vi "main_flow.vi"() -> ()   [LabVIEW 2022 SP3]
uses:
  D:/UOM/EE2044 - Electrical Measurements and Instrumentation/Project/Measurment Project/Quaxo_MQTT_LabVIEW-master/Controls/Connection_Return_Codes.ctl
  D:/UOM/EE2044 - Electrical Measurements and Instrumentation/Project/Measurment Project/Quaxo_MQTT_LabVIEW-master/Controls/QoS.ctl
  D:/UOM/EE2044 - Electrical Measurements and Instrumentation/Project/Measurment Project/Quaxo_MQTT_LabVIEW-master/Controls/Retain_Flag.ctl
  D:/UOM/EE2044 - Electrical Measurements and Instrumentation/Project/Measurment Project/Quaxo_MQTT_LabVIEW-master/Controls/DUP_Flag.ctl
  D:/UOM/EE2044 - Electrical Measurements and Instrumentation/Project/Measurment Project/Quaxo_MQTT_LabVIEW-master/Controls/Connect_Flags.ctl
  D:/UOM/EE2044 - Electrical Measurements and Instrumentation/Project/Measurment Project/Quaxo_MQTT_LabVIEW-master/Controls/User_Info.ctl
  <vilib>/DAQmx/write.llb/DAQmx Write (Digital Bool 1Line 1Point).vi
  <vilib>/DAQmx/read.llb/DAQmx Read (Digital Bool 1Line 1Point).vi
  <vilib>/DAQmx/read.llb/DAQmx Read (Analog 1D DBL NChan 1Samp).vi
  <vilib>/DAQmx/create/channels.llb/DAQmx Create Channel (AI-Voltage-Basic).vi
  <vilib>/DAQmx/create/channels.llb/DAQmx Create Channel (DO-Digital Output).vi
  <vilib>/DAQmx/create/channels.llb/DAQmx Create Channel (DI-Digital Input).vi
  <vilib>/DAQmx/miscellaneous.llb/DAQmx Fill In Error Info.vi
  D:/UOM/EE2044 - Electrical Measurements and Instrumentation/Project/Measurment Project/Quaxo_MQTT_LabVIEW-master/MQTT_Functions.lvlib
panel:
  out "Current":dbl(knob) caption="Current (A)" scale=0.0..5.0
  out "Energy":dbl caption="Energy( VA )"
  in  "clock stop":bool
  out "Time":string
  out "Servo Angle":dbl(knob) scale=0.0..150.0
  in  "stop (F)":bool
  out "PWM Wave":dynamicdata(graph) caption="Square"
  in  "Frequency":dbl=50.0
  in  "Offset":dbl=2.5
  in  "Amplitude":dbl=2.5
  in  "MQTT Broker":cluster{"address (IP)":string, "port":u16}={"address (IP)"="broker.mqttdashboard.com", "port"=1883}
  out "Counter":dbl
  out "OUT COUNT":dbl
  out "IN COUNT":dbl
  in  "Mode":dbl
  in  "Relay 2":tag
  in  "Relay 1":tag
  in  "UP DOWN 2":tag
  in  "UP DOWN 1":tag
  in  "Buzzer":tag
  in  "Door IR 1 & 2 & LDR & Current":tag
  out "LDR Value":dbl(knob) scale=0.0..5.0
  in  "Trigger Period(sec)":dbl
  out "?":bool
  out "?":bool
  out "?":bool
  in  "mqtt stop":bool
  in  "Publish Meta":cluster{"QoS":T1, "Retain":T2, "DUP":T3}
  out "Connection Status":T4=enum."Connection refused: not authorized"
  in  "Client ID":string="NodeE-12345"
  out "Current Time":dbl
  in  "stop":bool
  # "Channel Configure"
  # "MQTT Configure"
  # "MQTT publish interval\nset MQTT Server \nset channels\nset check mode trigger period"
  # "Dev1/ai4:7"
  # "Dev1/port0/line2"
  # "Dev1/port0/line1"
  # "broker.mqtt.cool"
  # "Dev1/port0/line0"
  # "Dev1/port0/line3"
  # "Servo Motor Controller"
  # "Energy Calculation"
  # "Dev1/port0/line4"
  # "Counter Status"
  # "Light Mode"
  # "Low"
  # "Medium"
  # "High"
  # "This Indicate the status of light mode in the room"
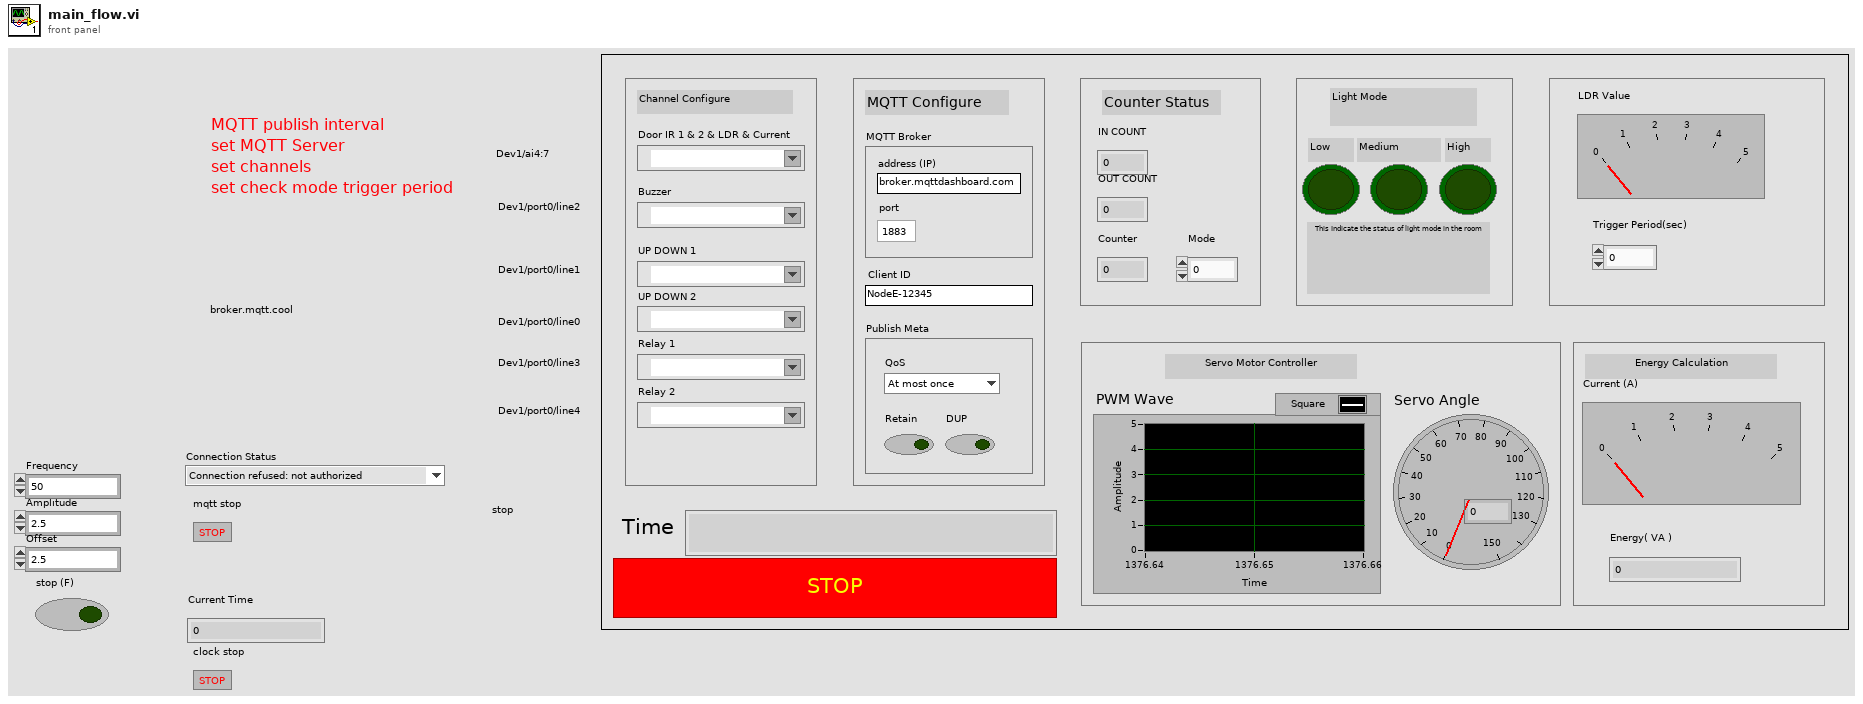
[diagram p1: front panel]
types:
  T1 = typedef "MQTT_Functions.lvlib/QoS.ctl" = enum8{"At most once", "At least once", "Exactly once", "Reserved"}
  T2 = typedef "MQTT_Functions.lvlib/Retain_Flag.ctl" = bool
  T3 = typedef "MQTT_Functions.lvlib/DUP_Flag.ctl" = bool
  T4 = typedef "MQTT_Functions.lvlib/Connection_Return_Codes.ctl" = enum16{"Connection accepted", "Connection refused: unacceptable protocol version", "Connection refused: identifier rejected", "Connection refused: Server unavailable", "Connection refused: bad user name or password", "Connection refused: not authorized"}
  T5 = typedef "MQTT_Functions.lvlib/User_Info.ctl" = cluster{"User Name":string, "Password":string}
  T6 = typedef "MQTT_Functions.lvlib/Connect_Flags.ctl" = cluster{"user name":bool, "password":bool, "will retain":bool, "will flag":bool, "clean session":bool, "reserved":bool, "will QoS":T1}
  T7 = cluster{"QoS":T1, "DUP":T3, "Retain":T2, "Keep Alive (sec)":u16}
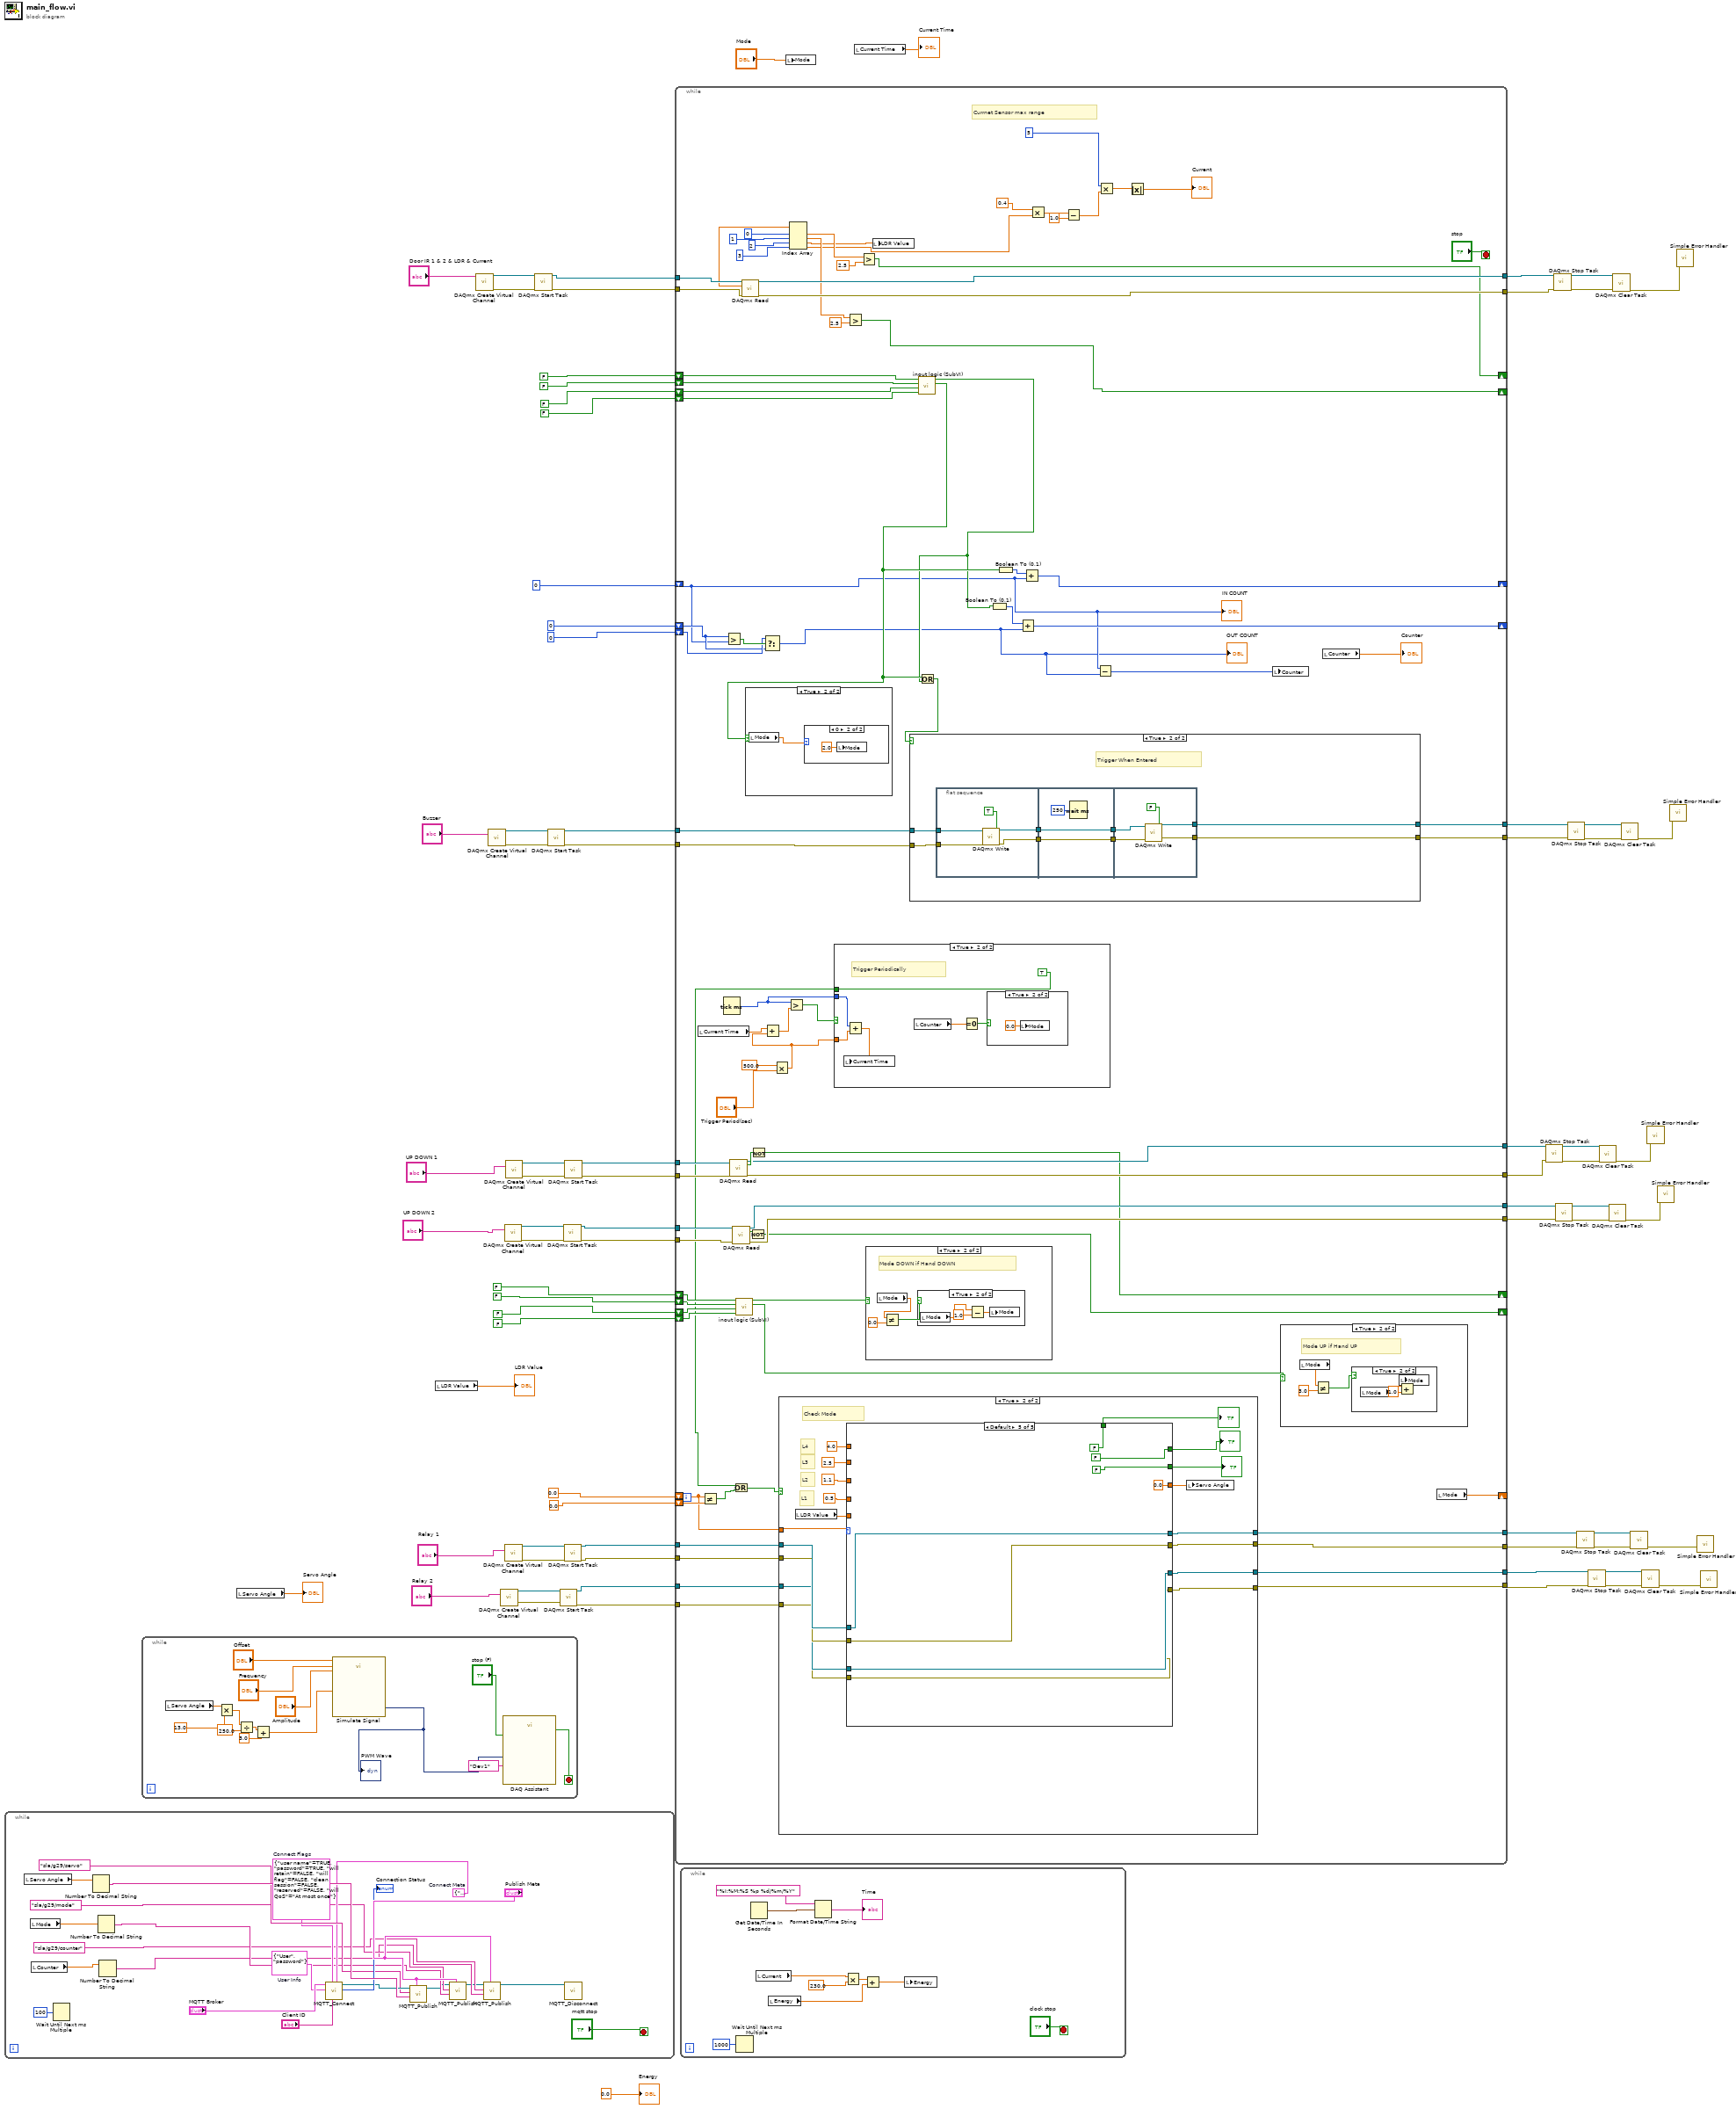
[diagram p0: block diagram]
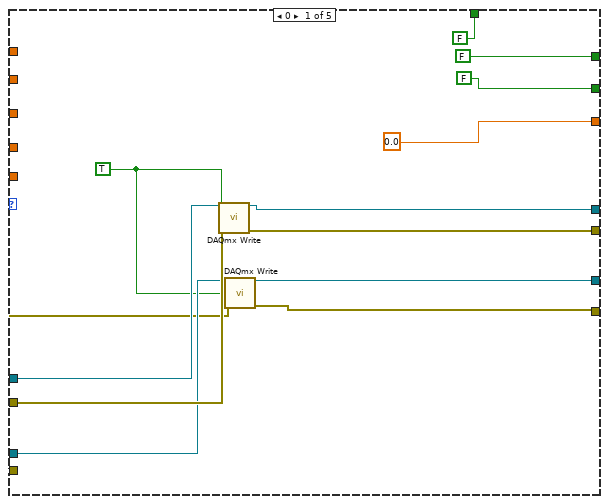
[diagram p5: hidden frame]
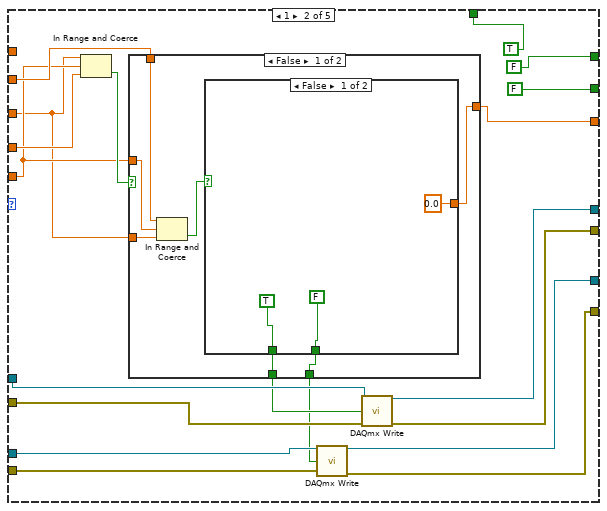
[diagram p6: hidden frame]
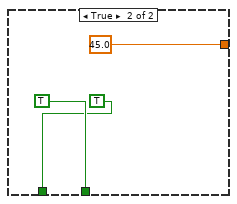
[diagram p7: hidden frame]
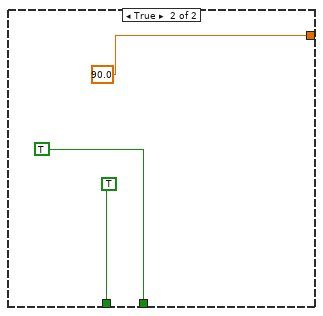
[diagram p8: hidden frame]
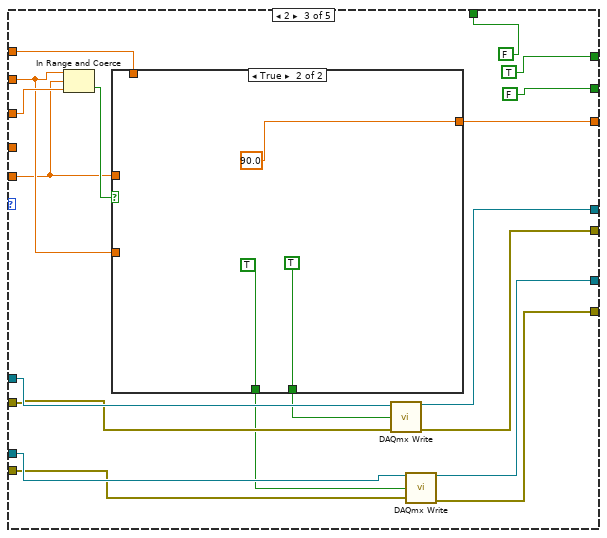
[diagram p9: hidden frame]
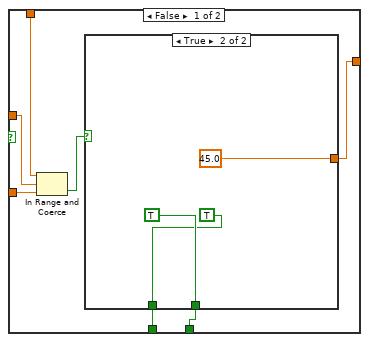
[diagram p10: hidden frame]
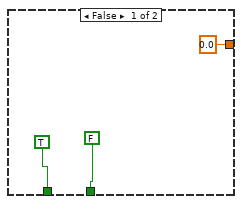
[diagram p11: hidden frame]
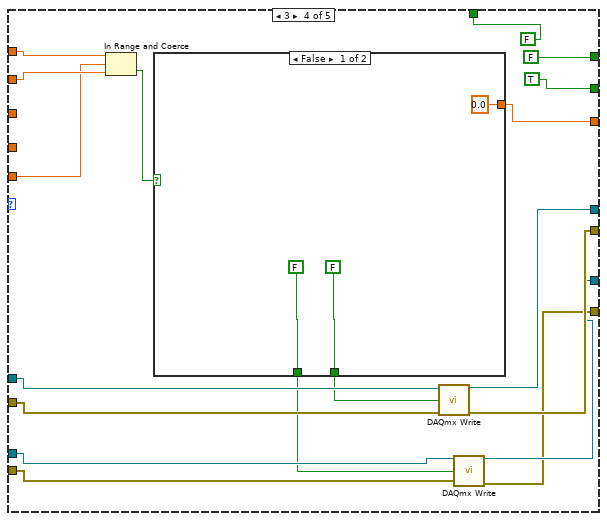
[diagram p12: hidden frame]
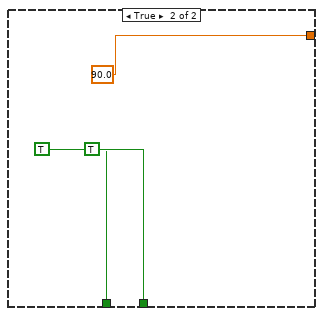
[diagram p13: hidden frame]
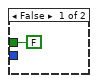
[diagram p18: hidden frame]
diagram:
  n1 = while {
    stop <- "mqtt stop" stop-if-true
    w86 = T5 {"User Name"="User", "Password"="password"}  # User Info
    w87 = T6 {"user name"=TRUE, "password"=TRUE, "will retain"=FALSE, "will flag"=FALSE, "clean session"=FALSE, "reserved"=FALSE, "will QoS"=enum."At most once"}  # Connect Flags
    w88 = T7 {"QoS"=enum."At most once", "DUP"=FALSE, "Retain"=FALSE, "Keep Alive (sec)"=60}  # Connect Meta
    n2 = local read "Servo Angle"() -> (w97:dbl)
    n3 = local read "Mode"() -> (w99:dbl)
    n4 = local read "Counter"() -> (w98:dbl)
    n5 = Wait Until Next ms Multiple(millisecond multiple=u32 100) -> ()  [unwired: 1 out]
    n6 = Number To Decimal String(number=w97) -> (decimal integer string=w96:string)  [unwired: 1 in]
    n7 = Number To Decimal String(number=w99) -> (decimal integer string=w85:string)  [unwired: 1 in]
    n8 = Number To Decimal String(number=w98) -> (decimal integer string=w83:string)  [unwired: 1 in]
    n9 = call "MQTT_Connect.vi"("Connect Meta"=w88, "Client ID"="Client ID", "Connect Flags"=w87, "User Info"=w86, "MQTT Broker"="MQTT Broker") -> ("Connection Status"=→"Connection Status":T4, "connection ID out"=w93:refnum<k5>)  [unwired: 4 in, 1 out]
    n10 = call "MQTT_Publish.vi"("Publish Meta"="Publish Meta", "Message to be published"=w96, "Topic"="sla/g29/servo", "connection ID"=w93) -> ("connection ID out"=w80:refnum<k5>)  [unwired: 6 in, 1 out]
    n11 = call "MQTT_Publish.vi"("Publish Meta"="Publish Meta", "Message to be published"=w85, "Topic"="sla/g29/mode", "connection ID"=w80) -> ("connection ID out"=w79:refnum<k5>)  [unwired: 6 in, 1 out]
    n12 = call "MQTT_Publish.vi"("Publish Meta"="Publish Meta", "Message to be published"=w83, "Topic"="sla/g29/counter", "connection ID"=w79) -> ("connection ID out"=w91:refnum<k5>)  [unwired: 6 in, 1 out]
    n13 = call "MQTT_Disconnect.vi"("connection ID"=w91) -> ()  [unwired: 10 in, 1 out]
  }
  n14 = while {
    stop <- w113 stop-if-true
    n15 = local read "Servo Angle"() -> (w101:dbl)
    n16 = Multiply(x=w101, y=13.0) -> (x*y=w107:dbl)
    n17 = Divide(x=w107, y=250.0) -> (x/y=w106:dbl)
    n18 = Add(x=w106, y=3.0) -> (x+y=w102:dbl)
    n19 = call "Simulate Signal"("Offset"="Offset", "Duty Cycle (%)"=w102, "Frequency"="Frequency", "Amplitude"="Amplitude") -> ("Square"=w109:dynamicdata)  [unwired: 10 in, 1 out]
    "PWM Wave" <- w109
    n20 = call "DAQ Assistant"("data"=w109, "stop (F)"="stop (F)", "device name"=tag "Dev1") -> ("stopped"=w113:bool)  [unwired: 14 in, 2 out]
  }
  n21 = local read "Servo Angle"() -> (→"Servo Angle":dbl)
  n22 = local read "LDR Value"() -> (→"LDR Value":dbl)
  n23 = call-poly <vilib>:"DAQmx Create Virtual Channel.vi"("physical channels"="Door IR 1 & 2 & LDR & Current") -> ("task out"=w74:refnum<k21>, "error out"=w71:errorcluster)  [unwired: 13 in]
  n24 = call-poly <vilib>:"DAQmx Create Virtual Channel.vi"("lines"="Buzzer") -> ("task out"=w59:refnum<k21>, "error out"=w57:errorcluster)  [unwired: 13 in]
  n25 = call-poly <vilib>:"DAQmx Create Virtual Channel.vi"("lines"="Relay 2") -> ("task out"=w20:refnum<k21>, "error out"=w19:errorcluster)  [unwired: 13 in]
  n26 = call-poly <vilib>:"DAQmx Create Virtual Channel.vi"("lines"="UP DOWN 2") -> ("task out"=w48:refnum<k21>, "error out"=w46:errorcluster)  [unwired: 13 in]
  n27 = call-poly <vilib>:"DAQmx Create Virtual Channel.vi"("lines"="Relay 1") -> ("task out"=w23:refnum<k21>, "error out"=w22:errorcluster)  [unwired: 13 in]
  n28 = call-poly <vilib>:"DAQmx Create Virtual Channel.vi"("lines"="UP DOWN 1") -> ("task out"=w49:refnum<k21>, "error out"=w47:errorcluster)  [unwired: 13 in]
  n29 = call <vilib>:"DAQmx Start Task.vi"("task/channels in"=w74, "error in"=w71) -> ("task out"=w72:refnum<k21>, "error out"=w70:errorcluster)  [unwired: 12 in]
  n30 = call <vilib>:"DAQmx Start Task.vi"("task/channels in"=w59, "error in"=w57) -> ("task out"=w56:refnum<k21>, "error out"=w55:errorcluster)  [unwired: 12 in]
  n31 = call <vilib>:"DAQmx Start Task.vi"("task/channels in"=w20, "error in"=w19) -> ("task out"=w15:refnum<k21>, "error out"=w14:errorcluster)  [unwired: 12 in]
  n32 = call <vilib>:"DAQmx Start Task.vi"("task/channels in"=w48, "error in"=w46) -> ("task out"=w41:refnum<k21>, "error out"=w40:errorcluster)  [unwired: 12 in]
  n33 = call <vilib>:"DAQmx Start Task.vi"("task/channels in"=w23, "error in"=w22) -> ("task out"=w17:refnum<k21>, "error out"=w16:errorcluster)  [unwired: 12 in]
  n34 = call <vilib>:"DAQmx Start Task.vi"("task/channels in"=w49, "error in"=w47) -> ("task out"=w43:refnum<k21>, "error out"=w42:errorcluster)  [unwired: 12 in]
  n35 = while {
    shift-right: [w192] -> _
    shift-left: 0.0 ("Mode") -> [w190]
    shift-left: 0.0 ("Mode") -> [w191]
    tunnel: w72 -> [w187]
    tunnel: w70 -> [w186]
    tunnel: [w185] -> w69
    tunnel: [w184] -> w68
    shift-right: [w116] -> _
    shift-left: FALSE -> [w183]
    shift-left: FALSE -> [w182]
    shift-right: [w115] -> _
    shift-left: FALSE -> [w181]
    shift-left: FALSE -> [w156]
    shift-right: [w180] -> _
    shift-left: 0 -> [w118]
    shift-right: [w179] -> _
    shift-left: 0 -> [w119]
    tunnel: w56 -> [w176]
    tunnel: w55 -> [w175]
    tunnel: [w174] -> w51
    tunnel: [w173] -> w50
    shift-right: [w162] -> _
    shift-left: FALSE -> [w160]
    shift-right: [w161] -> _
    shift-left: FALSE -> [w158]
    shift-left: FALSE -> [w159]
    shift-left: FALSE -> [w157]
    tunnel: w43 -> [w170]
    tunnel: w42 -> [w169]
    tunnel: w41 -> [w168]
    tunnel: w40 -> [w167]
    tunnel: [w166] -> w33
    tunnel: [w165] -> w32
    tunnel: [w164] -> w31
    tunnel: [w163] -> w30
    tunnel: w17 -> [w141]
    tunnel: w16 -> [w140]
    tunnel: w15 -> [w139]
    tunnel: w14 -> [w138]
    tunnel: [w137] -> w7
    tunnel: [w136] -> w6
    tunnel: [w135] -> w5
    tunnel: [w134] -> w4
    shift-left: 0 -> [w120]
    stop <- "stop" stop-if-true
    # "Currnet Sensor max range"
    n36 = local read "Current Time"() -> (w199:dbl)
    n37 = Not Equal?(x=w190, y=w191) -> (x != y?=w133:bool)
    n38 = Tick Count (ms)() -> (millisecond timer value=w197:u32)
    n39 = Greater?(x=w119, y=w118) -> (0:w121:bool)
    n40 = call-poly <vilib>:"DAQmx Read.vi"("task/channels in"=w170, "error in"=w169) -> ("task out"=w166:refnum<k21>, "data"=w172:bool, "error out"=w165:errorcluster)  [unwired: 11 in]
    n41 = call-poly <vilib>:"DAQmx Read.vi"("task/channels in"=w168, "error in"=w167) -> ("task out"=w164:refnum<k21>, "data"=w171:bool, "error out"=w163:errorcluster)  [unwired: 11 in]
    n42 = call "inout logic (SubVI).vi"("Sensor 2 (T-2)"=w157, "Sensor 2 (T-1)"=w158, "Sensor 1 (T-2)"=w159, "Sensor 1 (T-1)"=w160) -> ("IN"=w155:bool, "OUT"=w154:bool)  [unwired: 6 in]
    n43 = call-poly <vilib>:"DAQmx Read.vi"("task/channels in"=w187, "error in"=w186) -> ("task out"=w185:refnum<k21>, "data"=w151:dbl[], "error out"=w184:errorcluster)  [unwired: 11 in]
    n44 = Not(x=w171) -> (.not. x?=w161:bool)
    n45 = Not(x=w172) -> (.not. x?=w162:bool)
    n46 = Select(t=w120, s=w121, f=w119) -> (s? t:f=w117:i32)
    "OUT COUNT" <- w117
    n47 = Multiply(x=500.0, y="Trigger Period(sec)") -> (x*y=w193:dbl)
    n48 = Add(x=w199, y=w193) -> (x+y=w196:dbl)
    n49 = Greater?(x=w197, y=w196) -> (0:w198:bool)
    n50 = Index Array(array=w151, index #1=0 ("index"), index #2=1 ("index"), index #3=2 ("index"), index #4=3 ("index")) -> (element #1=w150:dbl, element #2=w147:dbl, element #3=w142:dbl, element #4=w124:dbl)
    n51 = case shown="True" w198 {
      tunnel: w197 -> [_ w357]
      tunnel: w193 -> [_ w356]
      tunnel: [FALSE ("Check") TRUE ("Check")] -> w131
      frame False {
      }
      frame True {
        # "Trigger Periodically"
        n52 = Add(x=w357, y=w356) -> (x+y=w358:dbl)
        n53 = local write "Current Time"(w358) -> ()
        n54 = local read "Counter"() -> (w355:dbl)
        n55 = Equal To 0?(x=w355) -> (x = 0?=w354:bool)
        n56 = case shown="True" w354 {
          frame False {
          }
          frame True {
            n57 = local write "Mode"(0.0 ("Mode")) -> ()
          }
        }
      }
    }
    n58 = Or(x=w131, y=w133) -> (x .or. y?=w132:bool)
    n59 = case shown="True" w132 {
      tunnel: w190 -> [_ w224]
      tunnel: w141 -> [w206 w223]
      tunnel: w140 -> [w205 w222]
      tunnel: w139 -> [w204 w221]
      tunnel: w138 -> [w203 w220]
      tunnel: [w206 w219] -> w137
      tunnel: [w205 w218] -> w136
      tunnel: [w204 w217] -> w135
      tunnel: [w203 w216] -> w134
      frame False {
      }
      frame True {
        # "L4"
        # "L1"
        # "L3"
        # "L2"
        # "Check Mode"
        n60 = local read "LDR Value"() -> (w214:dbl)
        n61 = case shown="Default" w224 {
          tunnel: w223 -> [w237 w256 w291 w325 w339]
          tunnel: w222 -> [w236 w254 w290 w324 w338]
          tunnel: w221 -> [w235 w252 w289 w323 w337]
          tunnel: w220 -> [w234 w250 w288 w322 w336]
          tunnel: [w233 w255 w287 w321 w339] -> w219
          tunnel: [w232 w253 w286 w320 w338] -> w218
          tunnel: [w231 w251 w285 w319 w337] -> w217
          tunnel: [w230 w249 w284 w318 w336] -> w216
          tunnel: 1.1 -> [_ w244 w283 _ _]
          tunnel: 0.5 -> [_ w247 _ _ _]
          tunnel: w214 -> [_ w245 w276 w314 _]
          tunnel: 2.5 -> [_ w246 w277 w315 _]
          tunnel: 4.0 -> [_ _ w278 w316 _]
          tunnel: [0.0 ("Servo Angle") w241 w281 w313 0.0 ("A")] -> w210
          tunnel: [FALSE TRUE FALSE FALSE FALSE] -> w209
          tunnel: [FALSE FALSE TRUE FALSE FALSE] -> w208
          tunnel: [FALSE FALSE FALSE TRUE FALSE] -> w207
          frame 0 {
            w229 = TRUE ("data")
            n62 = call-poly <vilib>:"DAQmx Write.vi"("task/channels in"=w237, "data"=w229, "error in"=w236) -> ("task out"=w233:refnum<k21>, "error out"=w232:errorcluster)  [unwired: 10 in, 1 out]
            n63 = call-poly <vilib>:"DAQmx Write.vi"("task/channels in"=w235, "data"=w229, "error in"=w234) -> ("task out"=w231:refnum<k21>, "error out"=w230:errorcluster)  [unwired: 10 in, 1 out]
          }
          frame 1 {
            n64 = In Range and Coerce(upper limit=w244, x=w245, lower limit=w247) -> (In Range?=w248:bool)  [unwired: 1 out]
            n65 = case shown="False" w248 {
              tunnel: [w259 90.0] -> w241
              tunnel: [w258 TRUE] -> w242
              tunnel: [w257 TRUE] -> w243
              tunnel: w246 -> [w263 _]
              tunnel: w244 -> [w262 _]
              tunnel: w245 -> [w261 _]
              frame False {
                n66 = In Range and Coerce(upper limit=w263, x=w261, lower limit=w262) -> (In Range?=w260:bool)  [unwired: 1 out]
                n67 = case shown="False" w260 {
                  tunnel: [0.0 45.0] -> w259
                  tunnel: [FALSE TRUE] -> w258
                  tunnel: [TRUE TRUE] -> w257
                  frame False {
                  }
                  frame True {
                  }
                }
              }
              frame True {
              }
            }
            n68 = call-poly <vilib>:"DAQmx Write.vi"("task/channels in"=w252, "data"=w242, "error in"=w250) -> ("task out"=w251:refnum<k21>, "error out"=w249:errorcluster)  [unwired: 10 in, 1 out]
            n69 = call-poly <vilib>:"DAQmx Write.vi"("task/channels in"=w256, "data"=w243, "error in"=w254) -> ("task out"=w255:refnum<k21>, "error out"=w253:errorcluster)  [unwired: 10 in, 1 out]
          }
          frame 2 {
            n70 = In Range and Coerce(upper limit=w277, x=w276, lower limit=w283) -> (In Range?=w282:bool)  [unwired: 1 out]
            n71 = case shown="True" w282 {
              tunnel: [w294 90.0] -> w281
              tunnel: [w293 TRUE] -> w280
              tunnel: [w292 TRUE] -> w279
              tunnel: w278 -> [w298 _]
              tunnel: w277 -> [w297 _]
              tunnel: w276 -> [w296 _]
              frame False {
                n72 = In Range and Coerce(upper limit=w298, x=w296, lower limit=w297) -> (In Range?=w295:bool)  [unwired: 1 out]
                n73 = case shown="True" w295 {
                  tunnel: [0.0 45.0] -> w294
                  tunnel: [FALSE TRUE] -> w293
                  tunnel: [TRUE TRUE] -> w292
                  frame False {
                  }
                  frame True {
                  }
                }
              }
              frame True {
              }
            }
            n74 = call-poly <vilib>:"DAQmx Write.vi"("task/channels in"=w291, "data"=w280, "error in"=w290) -> ("task out"=w287:refnum<k21>, "error out"=w286:errorcluster)  [unwired: 10 in, 1 out]
            n75 = call-poly <vilib>:"DAQmx Write.vi"("task/channels in"=w289, "data"=w279, "error in"=w288) -> ("task out"=w285:refnum<k21>, "error out"=w284:errorcluster)  [unwired: 10 in, 1 out]
          }
          frame 3 {
            n76 = In Range and Coerce(upper limit=w316, x=w314, lower limit=w315) -> (In Range?=w317:bool)  [unwired: 1 out]
            n77 = case shown="False" w317 {
              tunnel: [0.0 90.0] -> w313
              tunnel: [FALSE TRUE] -> w312
              tunnel: [FALSE TRUE] -> w311
              frame False {
              }
              frame True {
              }
            }
            n78 = call-poly <vilib>:"DAQmx Write.vi"("task/channels in"=w325, "data"=w312, "error in"=w324) -> ("task out"=w321:refnum<k21>, "error out"=w320:errorcluster)  [unwired: 10 in, 1 out]
            n79 = call-poly <vilib>:"DAQmx Write.vi"("task/channels in"=w323, "data"=w311, "error in"=w322) -> ("task out"=w319:refnum<k21>, "error out"=w318:errorcluster)  [unwired: 10 in, 1 out]
          }
          frame Default {
          }
        }
        "?" <- w207
        "?" <- w208
        "?" <- w209
        n80 = local write "Servo Angle"(w210) -> ()
      }
    }
    n81 = Greater?(x=w147, y=2.5) -> (0:w115:bool)
    n82 = Greater?(x=w150, y=2.5) -> (0:w116:bool)
    n83 = case shown="True" w154 {
      frame False {
      }
      frame True {
        # "Mode DOWN if Hand DOWN"
        n84 = local read "Mode"() -> (w342:dbl)
        n85 = Not Equal?(x=w342, y=0.0) -> (x != y?=w341:bool)
        n86 = case shown="True" w341 {
          frame False {
          }
          frame True {
            n87 = local read "Mode"() -> (w344:dbl)
            n88 = Subtract(x=w344, y=1.0) -> (x-y=w343:dbl)
            n89 = local write "Mode"(w343) -> ()
          }
        }
      }
    }
    n90 = local write "LDR Value"(w142) -> ()
    n91 = call "inout logic (SubVI).vi"("Sensor 2 (T-2)"=w156, "Sensor 2 (T-1)"=w181, "Sensor 1 (T-2)"=w182, "Sensor 1 (T-1)"=w183) -> ("IN"=w146:bool, "OUT"=w145:bool)  [unwired: 6 in]
    n92 = case shown="True" w146 {
      frame False {
      }
      frame True {
        n93 = local read "Mode"() -> (w201:dbl)
        n94 = case shown="0" w201 {
          frame Default {
          }
          frame 0 {
            n95 = local write "Mode"(2.0 ("Mode")) -> ()
          }
        }
      }
    }
    n96 = Or(x=w146, y=w145) -> (x .or. y?=w144:bool)
    n97 = case shown="True" w144 {
      tunnel: w176 -> [w360 w369]
      tunnel: w175 -> [w361 w368]
      tunnel: [w360 w363] -> w174
      tunnel: [w361 w362] -> w173
      frame False {
      }
      frame True {
        # "Trigger When Entered"
        n98 = flat-sequence {
          tunnel: w369 -> [w373]
          tunnel: w368 -> [w372]
          tunnel: [w371] -> w366
          tunnel: [w370] -> w364
          tunnel: [w376] -> w367
          tunnel: w366 -> [w376]
          tunnel: [w375] -> w365
          tunnel: w364 -> [w375]
          tunnel: w367 -> [w381]
          tunnel: w365 -> [w380]
          tunnel: [w379] -> w363
          tunnel: [w378] -> w362
          frame #0 {
            n99 = call-poly <vilib>:"DAQmx Write.vi"("task/channels in"=w373, "data"=TRUE, "error in"=w372) -> ("task out"=w371:refnum<k21>, "error out"=w370:errorcluster)  [unwired: 10 in, 1 out]
          }
          frame #1 {
            n100 = Wait (ms)(milliseconds to wait=u32 250) -> ()  [unwired: 1 out]
          }
          frame #2 {
            n101 = call-poly <vilib>:"DAQmx Write.vi"("task/channels in"=w381, "data"=FALSE, "error in"=w380) -> ("task out"=w379:refnum<k21>, "error out"=w378:errorcluster)  [unwired: 10 in, 1 out]
          }
        }
      }
    }
    n102 = Boolean To (0,1)(Boolean=w145) -> (0, 1=w188:i16)
    n103 = Boolean To (0,1)(Boolean=w146) -> (0, 1=w189:i16)
    n104 = Add(x=w188, y=w117) -> (x+y=w179:i32)
    n105 = Add(x=w189, y=w118) -> (x+y=w180:i32)
    n106 = Multiply(x=0.4, y=w124) -> (x*y=w129:dbl)
    n107 = Subtract(x=w129, y=1.0) -> (x-y=w127:dbl)
    n108 = Subtract(x=w118, y=w117) -> (x-y=w178:i32)
    n109 = Multiply(x=5, y=w127) -> (x*y=w123:dbl)
    n110 = Absolute Value(x=w123) -> (abs(x)=→"Current":dbl)
    n111 = local write "Counter"(w178) -> ()
    n112 = case shown="True" w155 {
      frame False {
      }
      frame True {
        # "Mode UP if Hand UP"
        n113 = local read "Mode"() -> (w348:dbl)
        n114 = Not Equal?(x=w348, y=3.0) -> (x != y?=w346:bool)
        n115 = case shown="True" w346 {
          frame False {
          }
          frame True {
            n116 = local read "Mode"() -> (w351:dbl)
            n117 = Add(x=w351, y=1.0) -> (x+y=w349:dbl)
            n118 = local write "Mode"(w349) -> ()
          }
        }
      }
    }
    n119 = local read "Counter"() -> (→"Counter":dbl)
    n120 = local read "Mode"() -> (w192:dbl)
    "IN COUNT" <- w118
  }
  n121 = while {
    stop <- "clock stop" stop-if-true
    n122 = Wait Until Next ms Multiple(millisecond multiple=u32 1000) -> ()  [unwired: 1 out]
    n123 = Get Date/Time In Seconds() -> (seconds since 1Jan1904=w392:timestamp)
    n124 = local read "Current"() -> (w385:dbl)
    n125 = local read "Energy"() -> (w384:dbl)
    n126 = Format Date/Time String(time format string (%c)="%I:%M:%S %p %d/%m/%Y", seconds (now)=w392) -> (date/time string=→"Time":string)  [unwired: 1 in]
    n127 = Multiply(x=w385, y=230.0) -> (x*y=w386:dbl)
    n128 = Add(x=w386, y=w384) -> (x+y=w383:dbl)
    n129 = local write "Energy"(w383) -> ()
  }
  n130 = local write "Mode"("Mode") -> ()
  n131 = local read "Current Time"() -> (→"Current Time":dbl)
  n132 = call <vilib>:"DAQmx Stop Task.vi"("task/channels in"=w33, "error in"=w32) -> ("task out"=w39:refnum<k21>, "error out"=w37:errorcluster)  [unwired: 12 in]
  n133 = call <vilib>:"DAQmx Stop Task.vi"("task/channels in"=w69, "error in"=w68) -> ("task out"=w67:refnum<k21>, "error out"=w66:errorcluster)  [unwired: 12 in]
  n134 = call <vilib>:"DAQmx Stop Task.vi"("task/channels in"=w31, "error in"=w30) -> ("task out"=w36:refnum<k21>, "error out"=w34:errorcluster)  [unwired: 12 in]
  n135 = call <vilib>:"DAQmx Stop Task.vi"("task/channels in"=w51, "error in"=w50) -> ("task out"=w54:refnum<k21>, "error out"=w52:errorcluster)  [unwired: 12 in]
  n136 = call <vilib>:"DAQmx Stop Task.vi"("task/channels in"=w7, "error in"=w6) -> ("task out"=w13:refnum<k21>, "error out"=w11:errorcluster)  [unwired: 12 in]
  n137 = call <vilib>:"DAQmx Stop Task.vi"("task/channels in"=w5, "error in"=w4) -> ("task out"=w10:refnum<k21>, "error out"=w8:errorcluster)  [unwired: 12 in]
  n138 = call <vilib>:"DAQmx Clear Task.vi"("task in"=w39, "error in"=w37) -> ("error out"=w38:errorcluster)  [unwired: 13 in]
  n139 = call <vilib>:"DAQmx Clear Task.vi"("task in"=w36, "error in"=w34) -> ("error out"=w35:errorcluster)  [unwired: 13 in]
  n140 = call <vilib>:"DAQmx Clear Task.vi"("task in"=w67, "error in"=w66) -> ("error out"=w65:errorcluster)  [unwired: 13 in]
  n141 = call <vilib>:"DAQmx Clear Task.vi"("task in"=w54, "error in"=w52) -> ("error out"=w53:errorcluster)  [unwired: 13 in]
  n142 = call <vilib>:"DAQmx Clear Task.vi"("task in"=w13, "error in"=w11) -> ("error out"=w12:errorcluster)  [unwired: 13 in]
  n143 = call <vilib>:"DAQmx Clear Task.vi"("task in"=w10, "error in"=w8) -> ("error out"=w9:errorcluster)  [unwired: 13 in]
  n144 = call <vilib>:"Simple Error Handler.vi"("error in (no error)"=w38) -> ()  [unwired: 4 in, 5 out]
  n145 = call <vilib>:"Simple Error Handler.vi"("error in (no error)"=w35) -> ()  [unwired: 4 in, 5 out]
  n146 = call <vilib>:"Simple Error Handler.vi"("error in (no error)"=w53) -> ()  [unwired: 4 in, 5 out]
  n147 = call <vilib>:"Simple Error Handler.vi"("error in (no error)"=w65) -> ()  [unwired: 4 in, 5 out]
  n148 = call <vilib>:"Simple Error Handler.vi"("error in (no error)"=w12) -> ()  [unwired: 4 in, 5 out]
  n149 = call <vilib>:"Simple Error Handler.vi"("error in (no error)"=w9) -> ()  [unwired: 4 in, 5 out]
  "Energy" <- 0.0 ("Energy")
